vi "CreateCurrentLogString.vi"(11 "Currents (A)":dbl[](array[numeric])) -> (3 "Currents Log String":string)   [LabVIEW 2012]
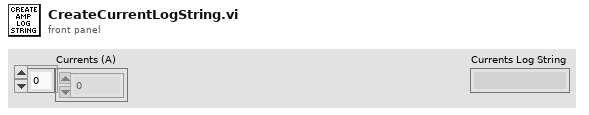
[diagram p1: front panel]
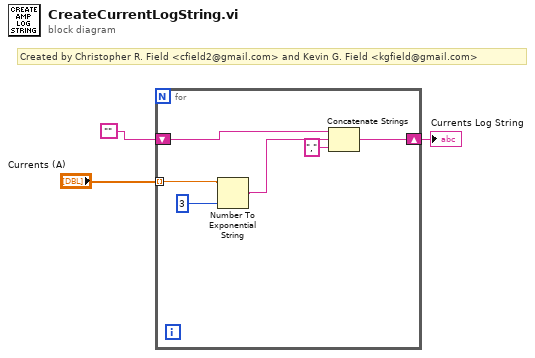
[diagram p0: block diagram]
diagram:
  # "Created by Christopher R. Field <cfield2@gmail.com> and Kevin G. Field <kgfield@gmail.com>"
  n1 = for {
    tunnel: "Currents (A)" -> [w6] mode=indexing
    shift-right: [w7] -> w1
    shift-left: "" -> [w9]
    n2 = Number To Exponential String(number=w6, precision (6)=i16 3) -> (E-format string=w5:string)  [unwired: 2 in]
    n3 = Concatenate Strings(w9, w5, "," ("string")) -> (w7:string)
  }
  "Currents Log String" <- w1
